vi "pp3_DAQ_AudioTriggerPlay.vi"(0 "Daq config In":T6={"Sound AO"="Dev6/ao0", "Shock intesity AO"="Dev6/ao1", "Code_LED DO"="Dev6/port1:2", "Switch DI"="Dev6/port1/line0", "Webcam"="cam9", "Sound AO task"="", "Sound card task"=0, "Shock intensity AO task"="", "Code_LED DO task"="", "Switch DI task"="", "AO <=> Sound card"=FALSE, "Sound card"=0, "sample rate"=100000.0, "Variable shock"=TRUE, "Webcam on"=FALSE, "Waveform memo"={"t0"=timestamp(0 s since 1904-01-01), "dt"=1.0, "Y"=[]}, "First time"=FALSE, "Tone trigger"="", "Master-9 DO"="Dev6/port0/line5:7"} {"sample rate" min=8000.0; "Sound card task" format="%.0x"}, 5 "State In":T1={"Curr  tr"=0, "Curr (ms)"=0, "Cum (ms)"=0, "Run loop diff"=0, "Tone countdown (ms)"=0, "Countdown (ms)"=0, "Curr State"=enum."0 NULL", "Prev State"=enum."1 Habituation", "Rw"=FALSE, "Sw"=FALSE, "Tone\nGate"=FALSE, "Punish"=FALSE, "Current DAQ DO Int"=0, "Current Loaded Trial"={"Trial Type Number"=1, "Trial Type"=enum."GO", "Trial Weight"=100, "Shock (mA)"=0.3, "Duration (ms)"=0.25, "Sound Type"=enum."04 FM Sweep", "Stim P1"=4000.0, "Stim P2"=0.0, "Stim P3"=0.0, "Stim P4"=2000.0, "DAQ Amplitude (V)"=0.25}, "Next Trial (for display purposes)"={"Trial Type Number"=1, "Trial Type"=enum."GO", "Trial Weight"=100, "Shock (mA)"=0.3, "Duration (ms)"=0.25, "Sound Type"=enum."04 FM Sweep", "Stim P1"=4000.0, "Stim P2"=0.0, "Stim P3"=0.0, "Stim P4"=2000.0, "DAQ Amplitude (V)"=0.25}, "Total trials memo"=0, "State start cum memo (ms)"=0, "Last dur jump time memo (ms)"=0, "Last dur shock time memo (ms)"=0, "Tone repeat memo (ms)"=0, "Webcam on"=FALSE, "Webcam recording"=FALSE, "State update flag"=FALSE, "Last loaded shock voltage"=0.0, "Vid upd"=enum."0"} {"Current DAQ DO Int" format="%016b"; "Next Trial (for display purposes)"."DAQ Amplitude (V)" min=0.0 max=5.0 format="%_4g"; "Next Trial (for display purposes)"."Shock (mA)" min=-1.0 max=5.0; "Next Trial (for display purposes)"."Trial Weight" step=1; "Next Trial (for display purposes)"."Duration (ms)" min=0.0 max=1.0; "Next Trial (for display purposes)"."Trial Type Number" min=1 max=256 step=1; "Current Loaded Trial"."DAQ Amplitude (V)" min=0.0 max=5.0 format="%_4g"; "Current Loaded Trial"."Shock (mA)" min=-1.0 max=5.0; "Current Loaded Trial"."Trial Weight" step=1; "Current Loaded Trial"."Duration (ms)" min=0.0 max=1.0; "Current Loaded Trial"."Trial Type Number" min=1 max=256 step=1}, 11 "error in (no error)":errorcluster) -> (4 "Daq config Out":T6={"Sound AO"="Dev6/ao0", "Shock intesity AO"="Dev6/ao1", "Code_LED DO"="Dev6/port1:2", "Switch DI"="Dev6/port1/line0", "Webcam"="cam9", "Sound AO task"="", "Sound card task"=0, "Shock intensity AO task"="", "Code_LED DO task"="", "Switch DI task"="", "AO <=> Sound card"=FALSE, "Sound card"=0, "sample rate"=100000.0, "Variable shock"=TRUE, "Webcam on"=FALSE, "Waveform memo"={"t0"=timestamp(0 s since 1904-01-01), "dt"=1.0, "Y"=[]}, "First time"=FALSE, "Tone trigger"="", "Master-9 DO"="Dev6/port0/line5:7"} {"sample rate" min=8000.0; "Sound card task" format="%.0x"}, 6 "State Out":T1={"Curr  tr"=0, "Curr (ms)"=0, "Cum (ms)"=0, "Run loop diff"=0, "Tone countdown (ms)"=0, "Countdown (ms)"=0, "Curr State"=enum."0 NULL", "Prev State"=enum."1 Habituation", "Rw"=FALSE, "Sw"=FALSE, "Tone\nGate"=FALSE, "Punish"=FALSE, "Current DAQ DO Int"=0, "Current Loaded Trial"={"Trial Type Number"=1, "Trial Type"=enum."GO", "Trial Weight"=100, "Shock (mA)"=0.3, "Duration (ms)"=0.25, "Sound Type"=enum."04 FM Sweep", "Stim P1"=4000.0, "Stim P2"=0.0, "Stim P3"=0.0, "Stim P4"=2000.0, "DAQ Amplitude (V)"=0.25}, "Next Trial (for display purposes)"={"Trial Type Number"=1, "Trial Type"=enum."GO", "Trial Weight"=100, "Shock (mA)"=0.3, "Duration (ms)"=0.25, "Sound Type"=enum."04 FM Sweep", "Stim P1"=4000.0, "Stim P2"=0.0, "Stim P3"=0.0, "Stim P4"=2000.0, "DAQ Amplitude (V)"=0.25}, "Total trials memo"=0, "State start cum memo (ms)"=0, "Last dur jump time memo (ms)"=0, "Last dur shock time memo (ms)"=0, "Tone repeat memo (ms)"=0, "Webcam on"=FALSE, "Webcam recording"=FALSE, "State update flag"=FALSE, "Last loaded shock voltage"=0.0, "Vid upd"=enum."0"} {"Current DAQ DO Int" format="%016b"; "Next Trial (for display purposes)"."DAQ Amplitude (V)" min=0.0 max=5.0 format="%_4g"; "Next Trial (for display purposes)"."Shock (mA)" min=-1.0 max=5.0; "Next Trial (for display purposes)"."Trial Weight" step=1; "Next Trial (for display purposes)"."Duration (ms)" min=0.0 max=1.0; "Next Trial (for display purposes)"."Trial Type Number" min=1 max=256 step=1; "Current Loaded Trial"."DAQ Amplitude (V)" min=0.0 max=5.0 format="%_4g"; "Current Loaded Trial"."Shock (mA)" min=-1.0 max=5.0; "Current Loaded Trial"."Trial Weight" step=1; "Current Loaded Trial"."Duration (ms)" min=0.0 max=1.0; "Current Loaded Trial"."Trial Type Number" min=1 max=256 step=1}, 15 "error out":errorcluster)   [LabVIEW 2013]
uses:
  pp3_CTL_DaqConfig.ctl
  <vilib>/userdefined/High Color/IMAQdx.ctl
  <vilib>/sound2/lvsound2.llb/Sound Output Task ID.ctl
  pp3_CTL_StateInfo.ctl
  pp3_CTL_State.ctl
  pp3_CTL_Trial.ctl
  pp3_CTL_TrialType.ctl
  labolabo2/waveforms/WFTypes.ctl
  <vilib>/sound2/lvsound2.llb/Sound Output Write (DBL Single).vi
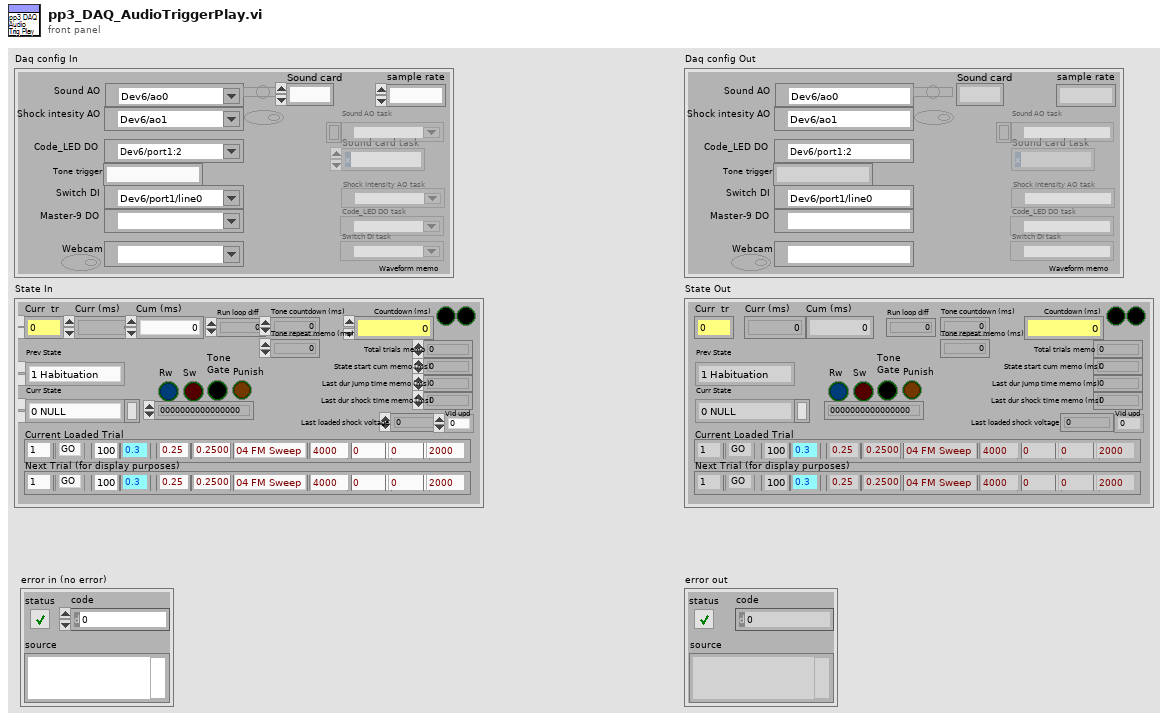
[diagram p1: front panel]
types:
  T1 = typedef "pp3_CTL_StateInfo.ctl" = cluster{"Curr  tr":u16, "Curr (ms)":u32, "Cum (ms)":i64, "Run loop diff":i64, "Tone countdown (ms)":i64, "Countdown (ms)":i64, "Curr State":T2, "Prev State":T2, "Rw":bool, "Sw":bool, "Tone\nGate":bool, "Punish":bool, "Current DAQ DO Int":u16, "Current Loaded Trial":T3, "Next Trial (for display purposes)":T3, "Total trials memo":i64, "State start cum memo (ms)":i64, "Last dur jump time memo (ms)":i64, "Last dur shock time memo (ms)":i64, "Tone repeat memo (ms)":i64, "Webcam on":bool, "Webcam recording":bool, "State update flag":bool, "Last loaded shock voltage":dbl, "Vid upd":enum16{"0", "1", "2", "3", "4", "5", "6", "7", "8", "9"}}
  T2 = typedef "pp3_CTL_State.ctl" = enum8{"0 NULL", "1 Habituation", "2 (Load Trial)", "3 Stay Period", "4 Load Audio/Click Delay", "5 GO Trial", "6 GO Jumped", "7 GO Timeout", "8 NOGO Trial", "9 NOGO Jumped", "10 NOGO Timeout", "11 TEST Trial", "12 TEST Jumped", "13 TEST Timeout", "14 Intertrial Interval", "15 Done"}
  T3 = typedef "pp3_CTL_Trial.ctl" = cluster{"Trial Type Number":i16, "Trial Type":T4, "Trial Weight":u32, "Shock (mA)":dbl, "Duration (ms)":dbl, "Sound Type":T5, "Stim P1":dbl, "Stim P2":dbl, "Stim P3":dbl, "Stim P4":dbl, "DAQ Amplitude (V)":dbl}
  T4 = typedef "pp3_CTL_TrialType.ctl" = enum16{"OFF", "GO", "NOGO", "TEST"}
  T5 = typedef "WFTypes.ctl" = enum16{"00 NULL", "01 DC", "02 Noise", "03 Pure Tone", "04 FM Sweep"}
  T6 = typedef "pp3_CTL_DaqConfig.ctl" = cluster{"Sound AO":tag, "Shock intesity AO":tag, "Code_LED DO":tag, "Switch DI":tag, "Webcam":T7, "Sound AO task":refnum<k21>, "Sound card task":T8, "Shock intensity AO task":refnum<k21>, "Code_LED DO task":refnum<k21>, "Switch DI task":refnum<k21>, "AO <=> Sound card":bool, "Sound card":u32, "sample rate":dbl, "Variable shock":bool, "Webcam on":bool, "Waveform memo":waveform(dbl), "First time":bool, "Tone trigger":string, "Master-9 DO":tag}
  T7 = typedef "IMAQdx.ctl" = refnum<k21>
  T8 = typedef "Sound Output Task ID.ctl" = u32
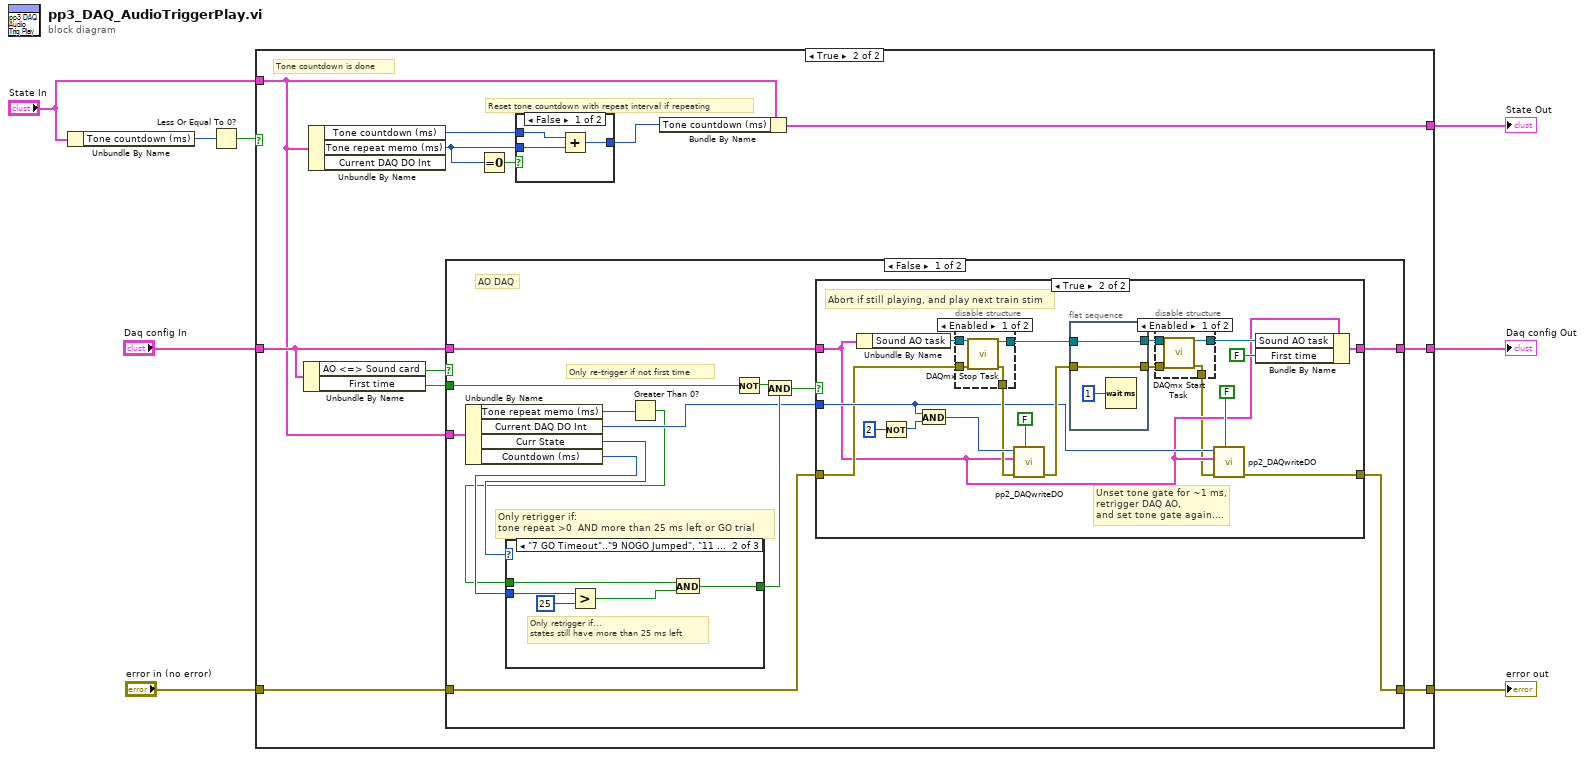
[diagram p0: block diagram]
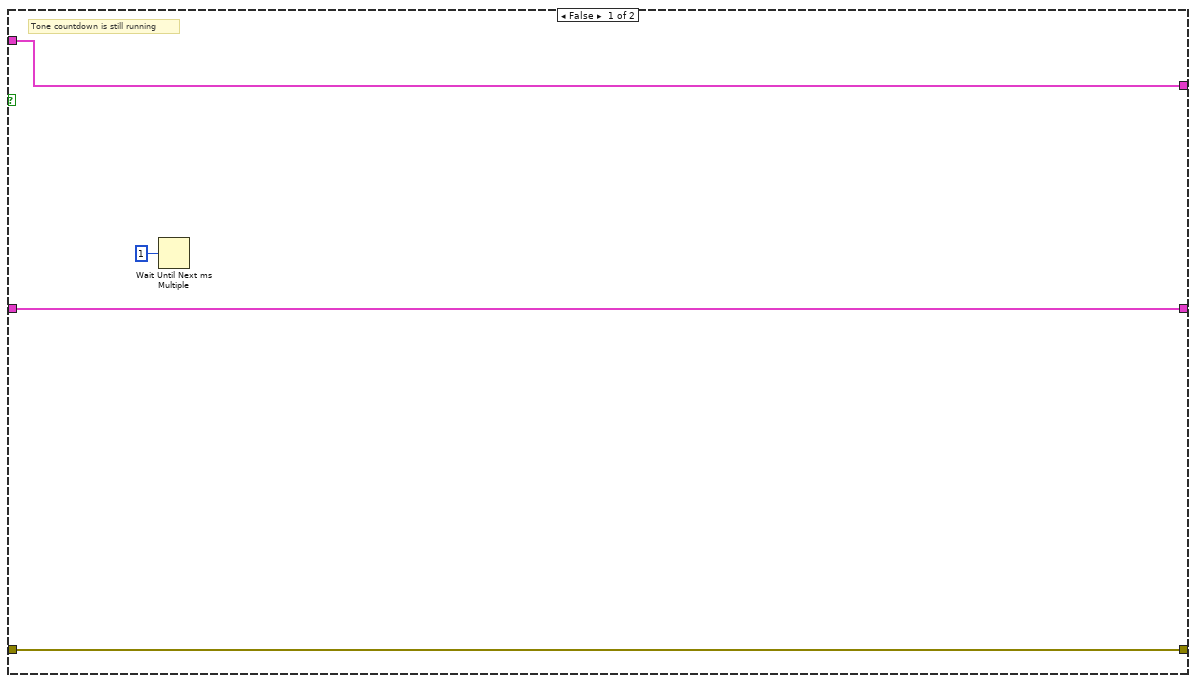
[diagram p2: hidden frame]
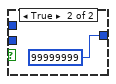
[diagram p3: hidden frame]
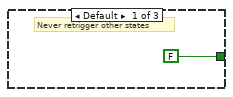
[diagram p4: hidden frame]
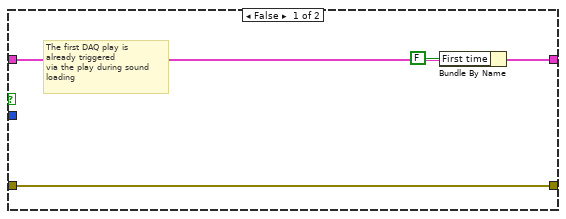
[diagram p6: hidden frame]
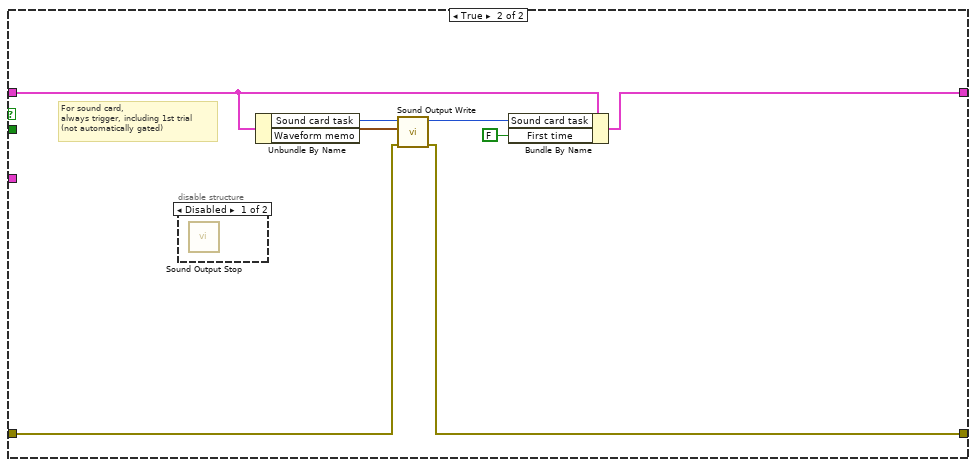
[diagram p9: hidden frame]
diagram:
  n1 = Unbundle By Name("State In") -> ("Tone countdown (ms)"=w4:i64)
  n2 = Less Or Equal To 0?(x=w4) -> (x <= 0?=w1:bool)
  n3 = case shown="True" w1 {
    tunnel: "Daq config In" -> [w12 w21]
    tunnel: [w12 w20] -> w7
    tunnel: "error in (no error)" -> [w11 w23]
    tunnel: [w11 w22] -> w5
    tunnel: "State In" -> [w9 w13]
    tunnel: [w9 w19] -> w2
    frame False {
      # "Tone countdown is still running"
      n4 = Wait Until Next ms Multiple(millisecond multiple=u32 1) -> ()  [unwired: 1 out]
    }
    frame True {
      # "Tone countdown is done"
      # "Reset tone countdown with repeat interval if repeating"
      n5 = Unbundle By Name(w21) -> ("AO <=> Sound card"=w24:bool, "First time"=w18:bool)
      n6 = Unbundle By Name(w13) -> ("Tone countdown (ms)"=w15:i64, "Tone repeat memo (ms)"=w16:i64)  [unwired: 1 out]
      n7 = case shown="False" w24 {
        tunnel: w23 -> [w35 w95]
        tunnel: [w42 w94] -> w22
        tunnel: w21 -> [w41 w92]
        tunnel: [w40 w93] -> w20
        tunnel: w18 -> [w29 _]
        tunnel: w13 -> [w39 _]
        frame False {
          # "Only retrigger if:\ntone repeat >0  AND more than 25 ms left or GO trial"
          # "Only re-trigger if not first time"
          # "AO DAQ"
          n8 = Unbundle By Name(w39) -> ("Tone repeat memo (ms)"=w31:i64, "Current DAQ DO Int"=w32:u16, "Curr State"=w34:T2, "Countdown (ms)"=w33:i64)
          n9 = Greater Than 0?(x=w31) -> (x > 0?=w30:bool)
          n10 = case shown="\"7 GO Timeout\"..\"9 NOGO Jumped\", \"11 TEST Trial\"" w34 {
            tunnel: [FALSE w46 w49] -> w36
            tunnel: w33 -> [_ w47 _]
            tunnel: w30 -> [_ w44 w49]
            frame Default {
              # "Never retrigger other states"
            }
            frame "7 GO Timeout".."9 NOGO Jumped", "11 TEST Trial" {
              # "Only retrigger if...\nstates still have more than 25 ms left"
              n11 = Greater?(x=w47, y=i64 25) -> (0:w45:bool)
              n12 = And(x=w44, y=w45) -> (x .and. y?=w46:bool)
            }
            frame "5 GO Trial" {
              # "GO Trial will always be retriggered\neven when less than 25 ms left,\nsince ending will lead to\ntone continuation and shock (miss)"
            }
          }
          n13 = Not(x=w29) -> (.not. x?=w37:bool)
          n14 = And(x=w37, y=w36) -> (x .and. y?=w38:bool)
          n15 = case shown="True" w38 {
            tunnel: w35 -> [w53 w62]
            tunnel: [w53 w66] -> w42
            tunnel: w41 -> [w51 w56]
            tunnel: [w50 w70] -> w40
            tunnel: w32 -> [_ w63]
            frame False {
              # "The first DAQ play is\nalready triggered\nvia the play during sound\nloading"
              n16 = Bundle By Name(cluster=w51, "First time"=FALSE) -> (w50:T6)
            }
            frame True {
              # "Abort if still playing, and play next train stim"
              # "Unset tone gate for ~1 ms,\nretrigger DAQ AO,\nand set tone gate again...."
              n17 = Unbundle By Name(w56) -> ("Sound AO task"=w71:refnum<k21>)
              n18 = Not(x=u16 2) -> (.not. x?=w68:u16)
              n19 = And(x=w63, y=w68) -> (x .and. y?=w67:u16)
              n20 = disable-structure shown="Enabled" {
                disable-tunnel: [w82 w84] -> w72
                disable-tunnel: w71 -> [w81 w84]
                disable-tunnel: [w80 w83] -> w65
                disable-tunnel: w62 -> [w79 w83]
                frame Enabled {
                  n21 = call <vilib>:"DAQmx Stop Task.vi"("task/channels in"=w81, "error in"=w79) -> ("task out"=w82:refnum<k21>, "error out"=w80:errorcluster)  [unwired: 12 in]
                }
                frame Disabled {
                }
              }
              n22 = call "pp2_DAQwriteDO.vi"("Reset to zero"=FALSE, "error in (no error)"=w65, "Daq config"=w56, "DAQ Digital In"=w67) -> ("error out"=w64:errorcluster)  [unwired: 7 in]
              n23 = flat-sequence {
                tunnel: w72 -> [w86]
                tunnel: [w85] -> w55
                tunnel: [w86] -> w58
                tunnel: w64 -> [w85]
                frame #0 {
                  n24 = Wait (ms)(milliseconds to wait=u32 1) -> ()  [unwired: 1 out]
                }
              }
              n25 = disable-structure shown="Enabled" {
                disable-tunnel: w58 -> [w76 w78]
                disable-tunnel: [w75 w78] -> w57
                disable-tunnel: w55 -> [w74 w77]
                disable-tunnel: [w73 w77] -> w54
                frame Enabled {
                  n26 = call <vilib>:"DAQmx Start Task.vi"("task/channels in"=w76, "error in"=w74) -> ("task out"=w75:refnum<k21>, "error out"=w73:errorcluster)  [unwired: 12 in]
                }
                frame Disabled {
                }
              }
              n27 = call "pp2_DAQwriteDO.vi"("Reset to zero"=FALSE, "error in (no error)"=w54, "Daq config"=w56, "DAQ Digital In"=w63) -> ("error out"=w66:errorcluster)  [unwired: 7 in]
              n28 = Bundle By Name(cluster=w56, "Sound AO task"=w57, "First time"=FALSE) -> (w70:T6)
            }
          }
        }
        frame True {
          # "For sound card,\nalways trigger, including 1st trial\n(not automatically gated)"
          n29 = disable-structure shown="Disabled" {
            frame Disabled {
              n30 = call <vilib>:"Sound Output Stop.vi"() -> ()  [unwired: 10 in, 2 out]
            }
            frame Enabled {
            }
          }
          n31 = Unbundle By Name(w92) -> ("Sound card task"=w91:T8, "Waveform memo"=w90:waveform(dbl))
          n32 = call-poly <vilib>:"Sound Output Write.vi"("error in (no error)"=w95, "data"=w90, "task ID"=w91) -> ("error out"=w94:errorcluster, "task ID out"=w89:T8)  [unwired: 7 in]
          n33 = Bundle By Name(cluster=w92, "Sound card task"=w89, "First time"=FALSE) -> (w93:T6)
        }
      }
      n34 = Equal To 0?(x=w16) -> (x = 0?=w17:bool)
      n35 = case shown="False" w17 {
        tunnel: w16 -> [w26 _]
        tunnel: w15 -> [w27 _]
        tunnel: [w25 i64 99999999] -> w14
        frame False {
          n36 = Add(x=w27, y=w26) -> (x+y=w25:i64)
        }
        frame True {
        }
      }
      n37 = Bundle By Name(cluster=w13, "Tone countdown (ms)"=w14) -> (w19:T1)
    }
  }
  "Daq config Out" <- w7
  "error out" <- w5
  "State Out" <- w2
